vi "Watch Circle Monitor (SubVI).vi"(7 "Queue in":refnum<queue>, 11 "GPS Source":enum16{"Spatial Dual", "V104", "XSens"}(ring)) -> (1 "Heading":string, 2 "Offset Distance":string, 3 "Current Position":string)   [LabVIEW 2019]
doc: "Monitors GPS position and calculates current offset from a configured set point in meters. Users can set watch circle radii in the Configurator and this function will generate alerts if the offset distance exceeds one or more radii. \n\n2021 NREL"
uses:
  Globals and Definitions/System Message.ctl
  bc948722-95b1-466d-8adc-bd7e1b37315f.vi
  Globals and Definitions/RT Globals RD v1.0.vi
  Globals and Definitions/Initialization Globals.vi
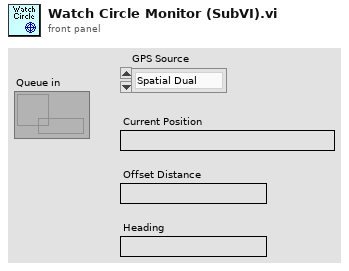
[diagram p1: front panel]
types:
  T1 = typedef "System Message.ctl" = cluster{"Message Tag":string, "Message Body":string, "Snooze Time (s)":dbl, "Snooze Alert?":bool, "Log Event?":bool, "Send Email":i32}
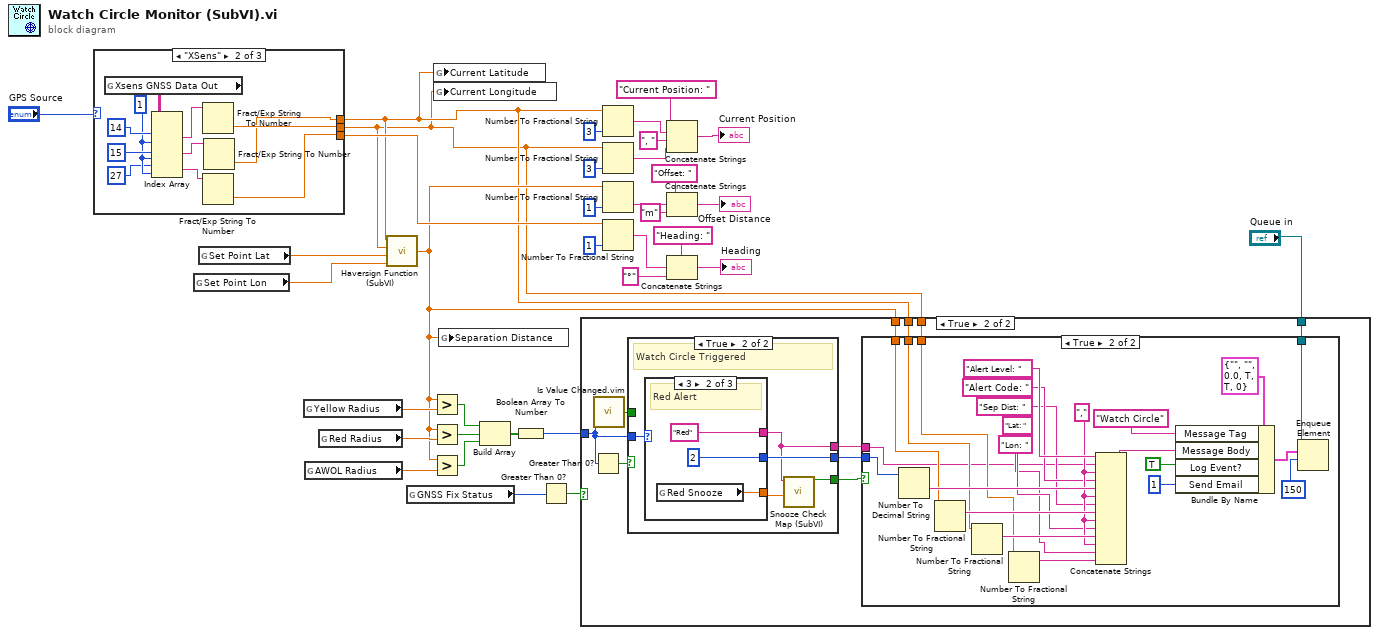
[diagram p0: block diagram]
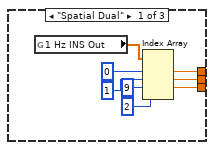
[diagram p2: hidden frame]
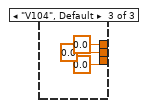
[diagram p3: hidden frame]
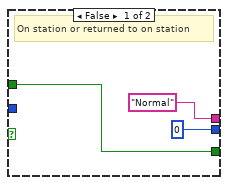
[diagram p5: hidden frame]
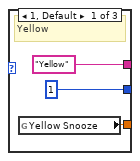
[diagram p6: hidden frame]
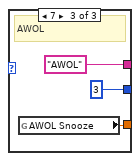
[diagram p7: hidden frame]
diagram:
  n1 = case shown="\"XSens\"" "GPS Source" {
    tunnel: [w42 w44 0.0 ("Height (m)")] -> w27
    tunnel: [w37 w48 0.0 ("Height (m)")] -> w4
    tunnel: [w36 w49 0.0 ("Height (m)")] -> w3
    frame "Spatial Dual" {
      n2 = global read "RT Globals RD v1.0.vi" "1 Hz INS Out"() -> (w38:dbl[])
      n3 = Index Array(array=w38, index #1=0 ("index"), index #2=1 ("index"), index #3=9 ("index"), index #4=2 ("index")) -> (element #1=w37:dbl, element #2=w36:dbl, element #3=w42:dbl)  [unwired: 1 out]
    }
    frame "XSens" {
      w47 = 1 ("disabled index (col)")
      n4 = global read "RT Globals RD v1.0.vi" "Xsens GNSS Data Out"() -> (w54:string[][])
      n5 = Index Array(array=w54, index (row) #1=14 ("index (row)"), index (col) #1=w47, index (row) #2=15 ("disabled index (row)"), index (col) #2=w47, index (row) #3=27 ("disabled index (row)"), index (col) #3=w47) -> (element #1=w51:string, element #2=w50:string, element #3=w45:string)
      n6 = Fract/Exp String To Number(string=w51) -> (number=w49:dbl)  [unwired: 3 in, 1 out]
      n7 = Fract/Exp String To Number(string=w45) -> (number=w44:dbl)  [unwired: 3 in, 1 out]
      n8 = Fract/Exp String To Number(string=w50) -> (number=w48:dbl)  [unwired: 3 in, 1 out]
    }
    frame "V104", Default {
    }
  }
  n9 = global read "Initialization Globals.vi" "Set Point Lon"() -> (w31:dbl)
  n10 = global read "Initialization Globals.vi" "Set Point Lat"() -> (w32:dbl)
  n11 = global read "Initialization Globals.vi" "Yellow Radius"() -> (w9:dbl)
  n12 = global read "Initialization Globals.vi" "AWOL Radius"() -> (w34:dbl)
  n13 = global read "Initialization Globals.vi" "Red Radius"() -> (w33:dbl)
  n14 = call "Haversign Function (SubVI).vi"("Set Point Lon (dd)"=w31, "Set Point Lat (dd)"=w32, "Current Lon (dd)"=w3, "Current Lat (dd)"=w4) -> ("Separation Distance (m)"=w5:dbl)
  n15 = global read "RT Globals RD v1.0.vi" "GNSS Fix Status"() -> (w2:u32)
  n16 = Greater?(x=w5, y=w9) -> (0:w8:bool)
  n17 = Greater?(x=w5, y=w33) -> (0:w28:bool)
  n18 = Greater?(x=w5, y=w34) -> (0:w29:bool)
  n19 = global write "RT Globals RD v1.0.vi" "Current Latitude"(w4) -> ()
  n20 = global write "RT Globals RD v1.0.vi" "Current Longitude"(w3) -> ()
  n21 = global write "RT Globals RD v1.0.vi" "Separation Distance"(w5) -> ()
  n22 = Build Array(w8, w28, w29) -> (w30:bool[])
  n23 = Boolean Array To Number(Boolean array=w30) -> (number=w7:u32)
  n24 = Greater Than 0?(x=w2) -> (x > 0?=w6:bool)
  n25 = case shown="True" w6 {
    tunnel: "Queue in" -> [_ w67]
    tunnel: w7 -> [_ w61]
    tunnel: w5 -> [_ w60]
    tunnel: w4 -> [_ w59]
    tunnel: w3 -> [_ w58]
    frame False {
    }
    frame True {
      n26 = Greater Than 0?(x=w61) -> (x > 0?=w66:bool)
      n27 = call "Is Value Changed.vim"("value"=w61) -> ("changed or first call?"=w65:bool)
      n28 = case shown="True" w66 {
        tunnel: ["Normal" ("WS Msg") w73] -> w63
        tunnel: [0 ("Alert Level") w75] -> w62
        tunnel: w61 -> [_ w74]
        tunnel: [w70 w71] -> w64
        tunnel: w65 -> [w70 _]
        frame False {
          # "On station or returned to on station"
        }
        frame True {
          # "Watch Circle Triggered"
          n29 = case shown="3" w74 {
            tunnel: [1 ("Alert Level") 2 ("Alert Level") 3 ("Alert Level")] -> w75
            tunnel: ["Yellow" ("WS Msg") "Red" ("WS Msg") "AWOL" ("WS Msg")] -> w73
            tunnel: [w76 w79 w82] -> w72
            frame 1, Default {
              # "Yellow"
              n30 = global read "Initialization Globals.vi" "Yellow Snooze"() -> (w76:dbl)
            }
            frame 3 {
              # "Red Alert"
              n31 = global read "Initialization Globals.vi" "Red Snooze"() -> (w79:dbl)
            }
            frame 7 {
              # "AWOL"
              n32 = global read "Initialization Globals.vi" "AWOL Snooze"() -> (w82:dbl)
            }
          }
          n33 = call "Snooze Check Map (SubVI).vi"("Snooze Time (s)"=w72, "key"=w73) -> ("Snooze Expired?"=w71:bool)  [unwired: 9 in]
        }
      }
      n34 = case shown="True" w64 {
        tunnel: w67 -> [_ w102]
        tunnel: w58 -> [_ w89]
        tunnel: w59 -> [_ w88]
        tunnel: w60 -> [_ w87]
        tunnel: w63 -> [_ w86]
        tunnel: w62 -> [_ w85]
        frame False {
        }
        frame True {
          w95 = ","
          n35 = Number To Decimal String(number=w85) -> (decimal integer string=w97:string)  [unwired: 1 in]
          n36 = Number To Fractional String(number=w87) -> (F-format string=w98:string)  [unwired: 3 in]
          n37 = Number To Fractional String(number=w88) -> (F-format string=w99:string)  [unwired: 3 in]
          n38 = Number To Fractional String(number=w89) -> (F-format string=w100:string)  [unwired: 3 in]
          n39 = Concatenate Strings("Alert Level: " ("Message Body"), w86, w95, "Alert Code: " ("Message Body"), w97, w95, "Sep Dist: " ("Message Body"), w98, w95, "Lat: " ("Message Body"), w99, w95, "Lon: " ("Message Body"), w100) -> (w90:string)
          n40 = Bundle By Name(cluster=T1 {"Message Tag"="", "Message Body"="", "Snooze Time (s)"=0.0, "Snooze Alert?"=TRUE, "Log Event?"=TRUE, "Send Email"=0}, "Message Tag"="Watch Circle", "Message Body"=w90, "Log Event?"=TRUE, "Send Email"=1) -> (w103:T1)
          n41 = Enqueue Element(queue=w102, element=w103, timeout in ms (-1)=150) -> ()  [unwired: 1 in, 3 out]
        }
      }
    }
  }
  n42 = Number To Fractional String(number=w4, precision (6)=i16 3) -> (F-format string=w12:string)  [unwired: 2 in]
  n43 = Number To Fractional String(number=w3, precision (6)=i16 3) -> (F-format string=w15:string)  [unwired: 2 in]
  n44 = Number To Fractional String(number=w5, precision (6)=i16 1) -> (F-format string=w23:string)  [unwired: 2 in]
  n45 = Number To Fractional String(number=w27, precision (6)=i16 1) -> (F-format string=w24:string)  [unwired: 2 in]
  n46 = Concatenate Strings("Current Position: " ("string"), w12, ", " ("string"), w15) -> (→"Current Position":string)
  n47 = Concatenate Strings("Offset: " ("string"), w23, "m" ("string")) -> (→"Offset Distance":string)
  n48 = Concatenate Strings("Heading: " ("string"), w24, "°" ("string")) -> (→"Heading":string)
